vi "User-defined Gate function.vi"(8 "Error In":errorcluster, 9 "User-defined Gate":T1, 11 "t":dbl format="%#_4g") -> (0 "Error Out":errorcluster, 3 "User-defined Gate(t)":dbl format="%#_4g")   [LabVIEW 2019]
doc: "Compute the value G(t) where t is the input time point and User-defined Gate is a cluster of two arrays, [t_i], i = 0, ..., n and [G_i}, i = 0,..., n as:\n1) G(t) = 0 if t < t_0 or t > t_n\n2) G(t) is linearly interpolated in between"
uses:
  Graphs/XY Graph/XY Plot Data.ctl
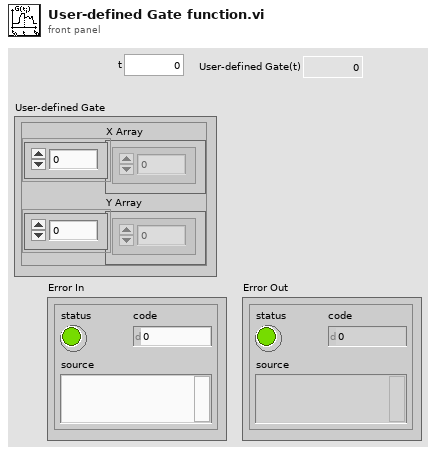
[diagram p1: front panel]
types:
  T1 = typedef "XY Plot Data.ctl" = cluster{"X Array":dbl[], "Y Array":dbl[]}
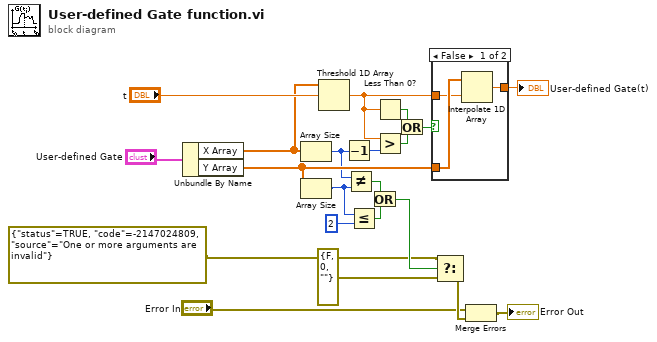
[diagram p0: block diagram]
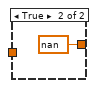
[diagram p2: hidden frame]
diagram:
  n1 = Unbundle By Name("User-defined Gate") -> ("X Array"=w19:dbl[], "Y Array"=w12:dbl[])
  n2 = Array Size(array=w19) -> (size(s)=w11:i32)
  n3 = Array Size(array=w12) -> (size(s)=w10:i32)
  n4 = Threshold 1D Array(2:"t", 3:w19) -> (0:w18:dbl)  [unwired: 1 in]
  n5 = Decrement(x=w11) -> (x-1=w14:i32)
  n6 = Not Equal?(x=w11, y=w10) -> (x != y?=w8:bool)
  n7 = Less Or Equal?(x=w10, y=2) -> (x <= y?=w7:bool)
  n8 = Or(x=w8, y=w7) -> (x .or. y?=w6:bool)
  n9 = Less Than 0?(x=w18) -> (x < 0?=w17:bool)
  n10 = Greater?(x=w18, y=w14) -> (0:w16:bool)
  n11 = Or(x=w17, y=w16) -> (x .or. y?=w15:bool)
  n12 = case shown="False" w15 {
    tunnel: w12 -> [w24 _]
    tunnel: [w23 nan] -> w20
    tunnel: w18 -> [w22 _]
    frame False {
      n13 = Interpolate 1D Array(1:w22, 2:w24) -> (0:w23:dbl)
    }
    frame True {
    }
  }
  "User-defined Gate(t)" <- w20
  n14 = Select(t=errorcluster {"status"=TRUE, "code"=-2147024809, "source"="One or more arguments are invalid"} ("error out"), s=w6, f=errorcluster {"status"=FALSE, "code"=0, "source"=""}) -> (s? t:f=w5:errorcluster)
  n15 = Merge Errors("Error In", w5) -> (→"Error Out":errorcluster)
